vi "Set Or get Row Head and Column Head Strings.vi"(7 "Row or Col Option":T1, 8 "error in (no error)":errorcluster caption="错误输入（无错误）", 9 "Mode":T2, 10 "Headers[] In":string[](array[string]), 11 "Table Ref In":refnum<vi>) -> (0 "error out":errorcluster caption="错误输出", 2 "Headers[] Out":string[](array[string]), 3 "Table Ref Out":refnum<vi>)   [LabVIEW 2012, in "Table Tool.lvlib"]
uses:
  Table Tool.lvlib
  GetOrSet.ctl
  Selet Row or Col.ctl
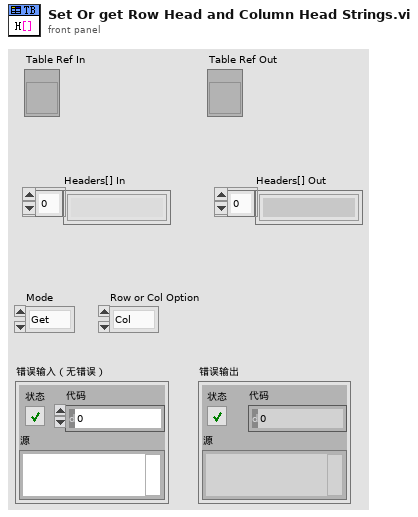
[diagram p1: front panel]
types:
  T1 = typedef "Table Tool.lvlib/Selet Row or Col.ctl" = enum16{"Col", "Row"}
  T2 = typedef "Table Tool.lvlib/GetOrSet.ctl" = enum16{"Get", "Set"}
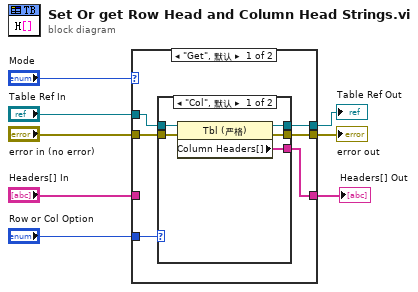
[diagram p0: block diagram]
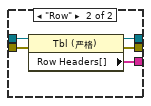
[diagram p2: hidden frame]
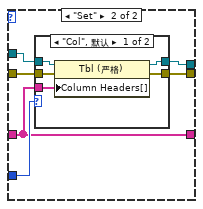
[diagram p3: hidden frame]
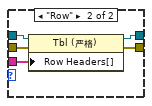
[diagram p4: hidden frame]
diagram:
  n1 = case shown="\"Get\", 默认" "Mode" {
    tunnel: "Table Ref In" -> [w13 w29]
    tunnel: "error in (no error)" -> [w14 w30]
    tunnel: [w11 w27] -> w5
    tunnel: [w12 w28] -> w4
    tunnel: "Row or Col Option" -> [w10 w26]
    tunnel: [w9 w25] -> w2
    tunnel: "Headers[] In" -> [_ w25]
    frame "Get", Default {
      n2 = case shown="\"Col\", 默认" w10 {
        tunnel: w14 -> [w17 w24]
        tunnel: w13 -> [w18 w23]
        tunnel: [w16 w22] -> w12
        tunnel: [w15 w21] -> w11
        tunnel: [w19 w20] -> w9
        frame "Col", Default {
          n3 = property class="Tbl (严格)"(reference=w18, error in=w17) -> (reference out=w16:refnum<vi>, error out=w15:errorcluster, "Column Headers[]"=w19:string[])
        }
        frame "Row" {
          n4 = property class="Tbl (严格)"(reference=w23, error in=w24) -> (reference out=w22:refnum<vi>, error out=w21:errorcluster, "Row Headers[]"=w20:string[])
        }
      }
    }
    frame "Set" {
      n5 = case shown="\"Col\", 默认" w26 {
        tunnel: w30 -> [w34 w40]
        tunnel: w29 -> [w33 w39]
        tunnel: [w31 w38] -> w28
        tunnel: [w32 w37] -> w27
        tunnel: w25 -> [w35 w36]
        frame "Col", Default {
          n6 = property class="Tbl (严格)"(reference=w33, error in=w34, "Column Headers[]"=w35) -> (reference out=w31:refnum<vi>, error out=w32:errorcluster)
        }
        frame "Row" {
          n7 = property class="Tbl (严格)"(reference=w39, error in=w40, "Row Headers[]"=w36) -> (reference out=w38:refnum<vi>, error out=w37:errorcluster)
        }
      }
    }
  }
  "Table Ref Out" <- w4
  "error out" <- w5
  "Headers[] Out" <- w2
